vi "Drive Controller.vi"(8 "error in":errorcluster) -> ()   [LabVIEW 2018]
doc: "This VI executes continuously carrying out the current operation and responding to updates or new operation requests. It will often contain the timing or control code that is difficult to place directly in TeleOp. This VI generally opens all sensors and motors and isolates the rest of the robot code from knowing implementation details of how the operations are carried out."
uses:
  <vilib>/Rock Robotics/WPI/Framework/Completion Status.ctl
  Drive Setpoints.ctl
  Drive Operations.ctl
  <vilib>/Rock Robotics/WPI/ThirdParty/Phoenix-LabVIEW/Motor Controller/Controls/CTRE_Phoenix_MotorControl_NeutralMode.ctl
  <vilib>/Rock Robotics/WPI/ThirdParty/Phoenix-LabVIEW/Motor Controller/Controls/CTRE_Phoenix_MotorControl_ControlMode.ctl
panel:
  in  "Interactive Values":T1
  in  "Buttons":cluster{"Execute Cmd":bool, "Abort Cmd":bool}
  out "Command Timing":cluster{"Start Time (ms)":u32, "Iterations":i32}
  out "Status":T3
  out "Current\nCmd":string
  # "Tip: The graph shows the motor setpoints. It may also be helpful to observe inputs and sensor values.\nYou may also want to display tuning or debugging controls."
  # "Interactive Command: You may fill in the settings for a command\nand schedule it with the Execute button. You can observe and abort\nany command while fine tuning the code for the controller."
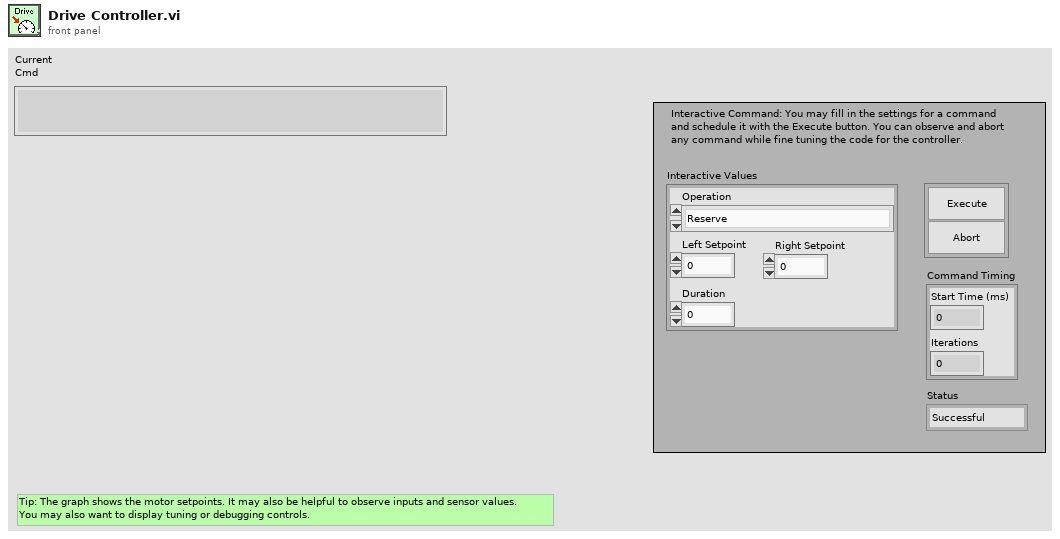
[diagram p1: front panel]
types:
  T1 = typedef "Drive Setpoints.ctl" = cluster{"Operation":T2, "Left Setpoint":dbl, "Right Setpoint":dbl, "Duration":dbl}
  T2 = typedef "Drive Operations.ctl" = enum16{"Reserve", "Read Current", "Immediate", "Drive for Time", "Drive for Distance"}
  T3 = typedef "Completion Status.ctl" = enum16{"Successful", "Aborted", "Incomplete"}
  T4 = typedef "CTRE_Phoenix_MotorControl_NeutralMode.ctl" = enum8{"EEPROMSetting", "Override to Coast", "Override to Brake"}
  T5 = enum16{"FollowerType_PercentOutput", "FollowerType_AuxOutput1"}
  T6 = typedef "WPI_MotorControlDeviceRef.ctl" = cluster{"DeviceStatus":errorcluster, "Type":T7, "PWM":cluster{"PWM Channel":T8, "DeadBand":T9}, "CAN":cluster{"Device Number":u8, "SetOutput VI Ref":variant, "GetOutput VI Ref":variant, "Enable VI Ref":variant, "Disable VI Ref":variant, "Data":variant}, "Invert":bool, "DIO PWM":cluster{"PWM \"Enable\" Channel":T8, "DIOChannel":T10, "PWM Rate":dbl}}
  T7 = typedef "WPI_MotorControlType.ctl" = enum16{"PWM", "CAN", "DIO PWM"}
  T8 = typedef "FPGA_DIOPWMChannel.ctl" = enum8{"PWM 0", "PWM 1", "PWM 2", "PWM 3", "PWM 4", "PWM 5", "PWM 6", "PWM 7", "PWM 8", "PWM 9", "PWM MXP 0", "PWM MXP 1", "PWM MXP 2", "PWM MXP 3", "PWM MXP 4", "PWM MXP 5", "PWM MXP 6", "PWM MXP 7", "PWM MXP 8", "PWM MXP 9", "Invalid"}
  T9 = typedef "WPI_PWMDeadband.ctl" = cluster{"Name":string, "maxPositivePwm":i32, "minPositivePwm":i32, "centerPwm":i32, "maxNegativePwm":i32, "minNegativePwm":i32, "angularRange":u16}
  T10 = typedef "FPGA_DIOChannel.ctl" = enum8{"DIO 0", "DIO 1", "DIO 2", "DIO 3", "DIO 4", "DIO 5", "DIO 6", "DIO 7", "DIO 8", "DIO 9", "DIO MXP 0", "DIO MXP 1", "DIO MXP 2", "DIO MXP 3", "DIO MXP 4", "DIO MXP 5", "DIO MXP 6", "DIO MXP 7", "DIO MXP 8", "DIO MXP 9", "DIO MXP 10", "DIO MXP 11", "DIO MXP 12", "DIO MXP 13", "DIO MXP 14", "DIO MXP 15", "SPI Port CS1", "SPI Port CS2", "SPI Port CS3", "SPI Port MISO", "SPI Port MOSI", "Invalid"}
  T11 = typedef "Command Status Info.ctl" = cluster{"Name":string, "Status":T3, "notifier out":T12}
  T12 = typedef "Completion Notifier.ctl" = refnum<notifier>
  T13 = cluster{"SubSystem Data":T1, cluster{"Start Time (ms)":u32, "Iterations":i32}, cluster{"Command Info":T11, "Description":string, "Default Command":T1, "queue out":refnum<queue>, "Subsystem Name":string}}
  T14 = enum16{"DemandType_Neutral", "DemandType_AuxPID", "DemandType_ArbitraryFeedForward"}
  T15 = typedef "CTRE_Phoenix_MotorControl_ControlMode.ctl" = u16
  T16 = cluster{"SubSystem Data":T1, cluster{"Start Time (ms)":u32, "Iterations":i32}, "Default Command Arguments":cluster{"Command Info":T11, "Description":string, "Default Command":T1, "queue out":refnum<queue>, "Subsystem Name":string}}
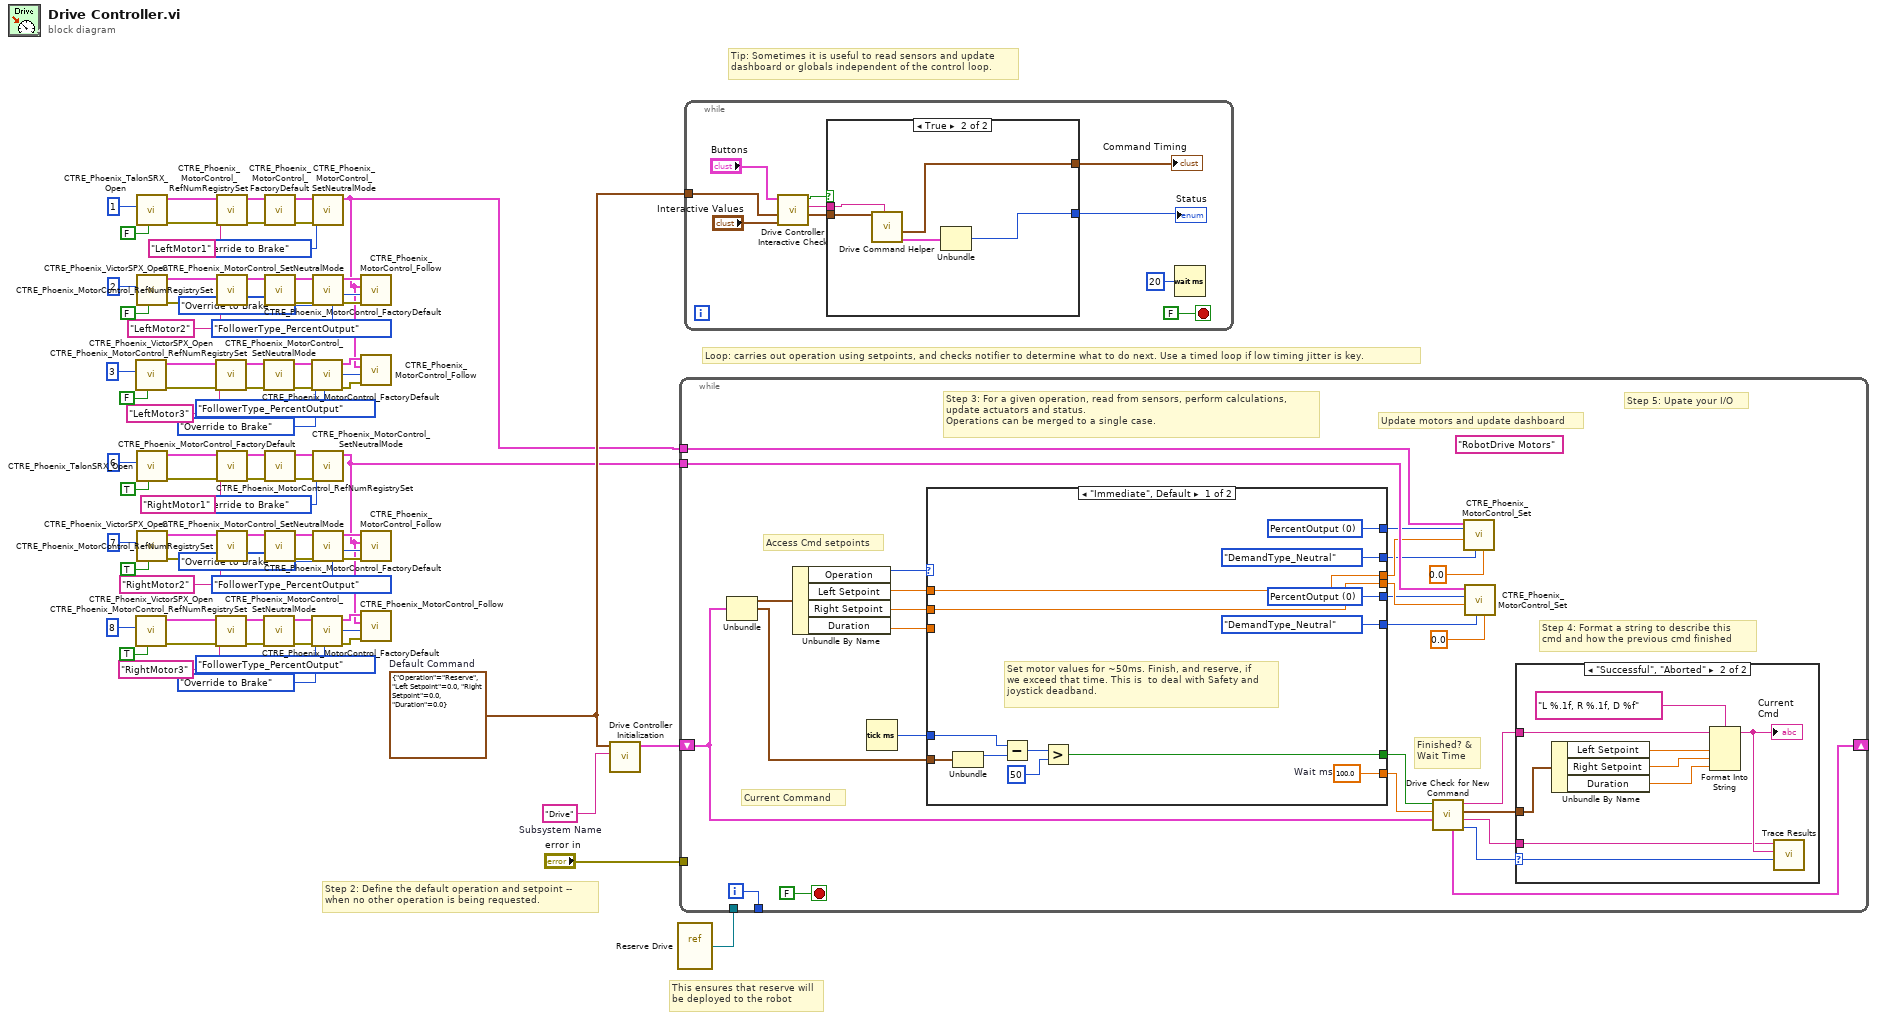
[diagram p0: block diagram]
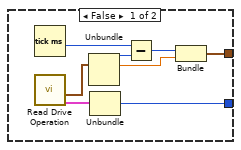
[diagram p2: hidden frame]
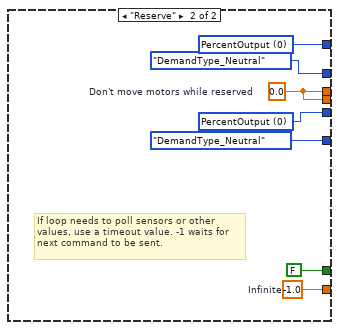
[diagram p4: hidden frame]
diagram:
  w75 = T1 {"Operation"=enum."Reserve", "Left Setpoint"=0.0, "Right Setpoint"=0.0, "Duration"=0.0}  # Default Command
  w79 = "Drive"  # Subsystem Name
  # "This ensures that reserve will\nbe deployed to the robot"
  # "Tip: Sometimes it is useful to read sensors and update\ndashboard or globals independent of the control loop."
  # "Step 2: Define the default operation and setpoint --\nwhen no other operation is being requested."
  # "Loop: carries out operation using setpoints, and checks notifier to determine what to do next. Use a timed loop if low timing jitter is key."
  n1 = call <vilib>:"CTRE_Phoenix_VictorSPX_Open.vi"("Invert"=FALSE, "Device Number"=u8 3) -> ("error out"=w48:errorcluster, "CAN Talon SRX Ref"=w49:T6)  [unwired: 8 in]
  n2 = call <vilib>:"CTRE_Phoenix_VictorSPX_Open.vi"("Invert"=TRUE, "Device Number"=u8 8) -> ("error out"=w12:errorcluster, "CAN Talon SRX Ref"=w13:T6)  [unwired: 8 in]
  n3 = call <vilib>:"CTRE_Phoenix_TalonSRX_Open.vi"("Invert"=FALSE, "Device Number"=u8 1) -> ("error out"=w68:errorcluster, "CAN Talon SRX Ref"=w74:T6)  [unwired: 8 in]
  n4 = call <vilib>:"CTRE_Phoenix_VictorSPX_Open.vi"("Invert"=FALSE, "Device Number"=u8 2) -> ("error out"=w57:errorcluster, "CAN Talon SRX Ref"=w58:T6)  [unwired: 8 in]
  n5 = call <vilib>:"CTRE_Phoenix_TalonSRX_Open.vi"("Invert"=TRUE, "Device Number"=u8 6) -> ("error out"=w32:errorcluster, "CAN Talon SRX Ref"=w38:T6)  [unwired: 8 in]
  n6 = call <vilib>:"CTRE_Phoenix_VictorSPX_Open.vi"("Invert"=TRUE, "Device Number"=u8 7) -> ("error out"=w21:errorcluster, "CAN Talon SRX Ref"=w22:T6)  [unwired: 8 in]
  n7 = call <vilib>:"CTRE_Phoenix_MotorControl_RefNumRegistrySet.vi"("error in (no error)"=w48, "refnum name"="LeftMotor3", "PhoenixMotorControlDevRef"=w49) -> ("error out"=w54:errorcluster, "PhoenixMotorControlDevRef"=w53:T6)  [unwired: 7 in]
  n8 = call <vilib>:"CTRE_Phoenix_MotorControl_RefNumRegistrySet.vi"("error in (no error)"=w12, "refnum name"="RightMotor3", "PhoenixMotorControlDevRef"=w13) -> ("error out"=w18:errorcluster, "PhoenixMotorControlDevRef"=w17:T6)  [unwired: 7 in]
  n9 = call <vilib>:"CTRE_Phoenix_MotorControl_RefNumRegistrySet.vi"("error in (no error)"=w68, "refnum name"="LeftMotor1", "PhoenixMotorControlDevRef"=w74) -> ("error out"=w70:errorcluster, "PhoenixMotorControlDevRef"=w69:T6)  [unwired: 7 in]
  n10 = call <vilib>:"CTRE_Phoenix_MotorControl_RefNumRegistrySet.vi"("error in (no error)"=w57, "refnum name"="LeftMotor2", "PhoenixMotorControlDevRef"=w58) -> ("error out"=w63:errorcluster, "PhoenixMotorControlDevRef"=w62:T6)  [unwired: 7 in]
  n11 = call <vilib>:"CTRE_Phoenix_MotorControl_RefNumRegistrySet.vi"("error in (no error)"=w32, "refnum name"="RightMotor1", "PhoenixMotorControlDevRef"=w38) -> ("error out"=w34:errorcluster, "PhoenixMotorControlDevRef"=w33:T6)  [unwired: 7 in]
  n12 = call <vilib>:"CTRE_Phoenix_MotorControl_RefNumRegistrySet.vi"("error in (no error)"=w21, "refnum name"="RightMotor2", "PhoenixMotorControlDevRef"=w22) -> ("error out"=w27:errorcluster, "PhoenixMotorControlDevRef"=w26:T6)  [unwired: 7 in]
  n13 = call <vilib>:"CTRE_Phoenix_MotorControl_FactoryDefault.vi"("error in"=w54, "PhoenixMotorControlDevRef"=w53) -> ("error out"=w52:errorcluster, "PhoenixMotorControlDevRef"=w51:T6)  [unwired: 8 in]
  n14 = call <vilib>:"CTRE_Phoenix_MotorControl_FactoryDefault.vi"("error in"=w18, "PhoenixMotorControlDevRef"=w17) -> ("error out"=w16:errorcluster, "PhoenixMotorControlDevRef"=w15:T6)  [unwired: 8 in]
  n15 = call <vilib>:"CTRE_Phoenix_MotorControl_FactoryDefault.vi"("error in"=w70, "PhoenixMotorControlDevRef"=w69) -> ("error out"=w67:errorcluster, "PhoenixMotorControlDevRef"=w66:T6)  [unwired: 8 in]
  n16 = call <vilib>:"CTRE_Phoenix_MotorControl_FactoryDefault.vi"("error in"=w63, "PhoenixMotorControlDevRef"=w62) -> ("error out"=w61:errorcluster, "PhoenixMotorControlDevRef"=w60:T6)  [unwired: 8 in]
  n17 = call <vilib>:"CTRE_Phoenix_MotorControl_FactoryDefault.vi"("error in"=w34, "PhoenixMotorControlDevRef"=w33) -> ("error out"=w31:errorcluster, "PhoenixMotorControlDevRef"=w30:T6)  [unwired: 8 in]
  n18 = call <vilib>:"CTRE_Phoenix_MotorControl_FactoryDefault.vi"("error in"=w27, "PhoenixMotorControlDevRef"=w26) -> ("error out"=w25:errorcluster, "PhoenixMotorControlDevRef"=w24:T6)  [unwired: 8 in]
  n19 = call <vilib>:"CTRE_Phoenix_MotorControl_SetNeutralMode.vi"("error in (no error)"=w52, "Motor Control Neutral Mode"=CTRE_Phoenix_MotorControl_NeutralMode."Override to Brake", "PhoenixMotorControlDevRef"=w51) -> ("error out"=w45:errorcluster, "PhoenixMotorControlDevRef"=w44:T6)  [unwired: 7 in]
  n20 = call <vilib>:"CTRE_Phoenix_MotorControl_SetNeutralMode.vi"("error in (no error)"=w16, "Motor Control Neutral Mode"=CTRE_Phoenix_MotorControl_NeutralMode."Override to Brake", "PhoenixMotorControlDevRef"=w15) -> ("error out"=w9:errorcluster, "PhoenixMotorControlDevRef"=w8:T6)  [unwired: 7 in]
  n21 = call <vilib>:"CTRE_Phoenix_MotorControl_SetNeutralMode.vi"("error in (no error)"=w67, "Motor Control Neutral Mode"=CTRE_Phoenix_MotorControl_NeutralMode."Override to Brake", "PhoenixMotorControlDevRef"=w66) -> ("PhoenixMotorControlDevRef"=w2:T6)  [unwired: 7 in, 1 out]
  n22 = call <vilib>:"CTRE_Phoenix_MotorControl_SetNeutralMode.vi"("error in (no error)"=w61, "Motor Control Neutral Mode"=CTRE_Phoenix_MotorControl_NeutralMode."Override to Brake", "PhoenixMotorControlDevRef"=w60) -> ("error out"=w47:errorcluster, "PhoenixMotorControlDevRef"=w46:T6)  [unwired: 7 in]
  n23 = call <vilib>:"CTRE_Phoenix_MotorControl_SetNeutralMode.vi"("error in (no error)"=w31, "Motor Control Neutral Mode"=CTRE_Phoenix_MotorControl_NeutralMode."Override to Brake", "PhoenixMotorControlDevRef"=w30) -> ("PhoenixMotorControlDevRef"=w1:T6)  [unwired: 7 in, 1 out]
  n24 = call <vilib>:"CTRE_Phoenix_MotorControl_SetNeutralMode.vi"("error in (no error)"=w25, "Motor Control Neutral Mode"=CTRE_Phoenix_MotorControl_NeutralMode."Override to Brake", "PhoenixMotorControlDevRef"=w24) -> ("error out"=w11:errorcluster, "PhoenixMotorControlDevRef"=w10:T6)  [unwired: 7 in]
  n25 = call <vilib>:"CTRE_Phoenix_MotorControl_Follow.vi"("error in (no error)"=w47, "FollowerType"=T5."FollowerType_PercentOutput", "Master Controller to Follow"=w2, "PhoenixMotorControlDevRef"=w46) -> ()  [unwired: 6 in, 2 out]
  n26 = call <vilib>:"CTRE_Phoenix_MotorControl_Follow.vi"("error in (no error)"=w45, "FollowerType"=T5."FollowerType_PercentOutput", "Master Controller to Follow"=w2, "PhoenixMotorControlDevRef"=w44) -> ()  [unwired: 6 in, 2 out]
  n27 = call <vilib>:"CTRE_Phoenix_MotorControl_Follow.vi"("error in (no error)"=w11, "FollowerType"=T5."FollowerType_PercentOutput", "Master Controller to Follow"=w1, "PhoenixMotorControlDevRef"=w10) -> ()  [unwired: 6 in, 2 out]
  n28 = call <vilib>:"CTRE_Phoenix_MotorControl_Follow.vi"("error in (no error)"=w9, "FollowerType"=T5."FollowerType_PercentOutput", "Master Controller to Follow"=w1, "PhoenixMotorControlDevRef"=w8) -> ()  [unwired: 6 in, 2 out]
  n29 = call "Drive Controller Initialization.vi"("Subsystem Name"=w79, "Default Command"=w75) -> ("Current Command"=w77:T13)  [unwired: 9 in]
  n30 = vi-ref "Reserve Drive.vi"() -> (w76:refnum<vi>)
  n31 = while {
    shift-right: [w97] -> _
    shift-left: w77 -> [w90]
    tunnel: [w105] -> _
    tunnel: "error in" -> [_]
    tunnel: w76 -> [_]
    tunnel: w2 -> [w89]
    tunnel: w1 -> [w88]
    i -> [w105]
    stop <- FALSE stop-if-true
    (unwired) "RobotDrive Motors" ("Name")
    # "Step 5: Upate your I/O"
    # "Step 4: Format a string to describe this\ncmd and how the previous cmd finished"
    # "Current Command"
    # "Update motors and update dashboard"
    # "Access Cmd setpoints"
    # "Finished? &\nWait Time"
    # "Step 3: For a given operation, read from sensors, perform calculations,\nupdate actuators and status.\nOperations can be merged to a single case."
    n32 = Unbundle(w90) -> ("SubSystem Data"=w104:T1, w91:cluster{"Start Time (ms)":u32, "Iterations":i32})  [unwired: 1 out]
    n33 = Unbundle By Name(w104) -> ("Operation"=w103:T2, "Left Setpoint"=w102:dbl, "Right Setpoint"=w101:dbl, "Duration"=w100:dbl)
    n34 = Tick Count (ms)() -> (millisecond timer value=w99:u32)
    n35 = case shown="\"Immediate\", Default" w103 {
      tunnel: [w128 w135] -> w96
      tunnel: [w121 FALSE ("ignore previous (F)")] -> w95
      tunnel: w91 -> [w120 _]
      tunnel: [w127 w133] -> w87
      tunnel: [w126 w133] -> w86
      tunnel: w102 -> [w127 _]
      tunnel: w101 -> [w126 _]
      tunnel: w100 -> [_ _]
      tunnel: w99 -> [w122 _]
      tunnel: [w117 w132] -> w85
      tunnel: [w119 w131] -> w84
      tunnel: [T14."DemandType_Neutral" ("DemandType") T14."DemandType_Neutral" ("DemandType")] -> w83
      tunnel: [T14."DemandType_Neutral" ("DemandType") T14."DemandType_Neutral" ("DemandType")] -> w82
      frame "Immediate", Default {
        w117 = T15 0 items=["PercentOutput"=0, "Position"=1, "Velocity"=2, "Current"=3, "Follower"=5, "MotionProfile"=6, "MotionMagic"=7, "MotionProfileArc"=10, "Disabled"=15] ("Control Mode")
        w119 = T15 0 items=["PercentOutput"=0, "Position"=1, "Velocity"=2, "Current"=3, "Follower"=5, "MotionProfile"=6, "MotionMagic"=7, "MotionProfileArc"=10, "Disabled"=15] ("Control Mode")
        w128 = 100.0  # Wait ms
        # "Set motor values for ~50ms. Finish, and reserve, if\nwe exceed that time. This is  to deal with Safety and\njoystick deadband."
        n36 = Unbundle(w120) -> ("Start Time (ms)"=w123:u32)  [unwired: 1 out]
        n37 = Subtract(x=w122, y=w123) -> (x-y=w124:u32)
        n38 = Greater?(x=w124, y=u8 50 ("Left Motor")) -> (0:w121:bool)
      }
      frame "Reserve" {
        w131 = T15 0 items=["PercentOutput"=0, "Position"=1, "Velocity"=2, "Current"=3, "Follower"=5, "MotionProfile"=6, "MotionMagic"=7, "MotionProfileArc"=10, "Disabled"=15] ("Control Mode")
        w132 = T15 0 items=["PercentOutput"=0, "Position"=1, "Velocity"=2, "Current"=3, "Follower"=5, "MotionProfile"=6, "MotionMagic"=7, "MotionProfileArc"=10, "Disabled"=15] ("Control Mode")
        w133 = 0.0  # Don't move motors while reserved
        w135 = -1.0  # Infinite
        # "If loop needs to poll sensors or other\nvalues, use a timeout value. -1 waits for\nnext command to be sent."
      }
    }
    n39 = call "Drive Check for New Command.vi"("input cluster"=w90, "Wait time (ms)"=w96, "Finished?"=w95) -> ("Completion"=w98:T3, "Subsystem Name"=w92:string, "Current Command"=w93:T1, "Initial Trace String"=w94:string, "Next Command"=w97:T16)  [unwired: 4 in]
    n40 = call <vilib>:"CTRE_Phoenix_MotorControl_Set.vi"("Demand1"=0.0, "DemandType"=w83, "Output"=w87, "Control Mode"=w84, "PhoenixMotorControlDevRef"=w89) -> ()  [unwired: 5 in, 2 out]
    n41 = call <vilib>:"CTRE_Phoenix_MotorControl_Set.vi"("Demand1"=0.0, "DemandType"=w82, "Output"=w86, "Control Mode"=w85, "PhoenixMotorControlDevRef"=w88) -> ()  [unwired: 5 in, 2 out]
    n42 = case shown="\"Successful\", \"Aborted\"" w98 {
      selector: w98 -> [_ w115]
      tunnel: w94 -> [_ w110]
      tunnel: w93 -> [_ w111]
      tunnel: w92 -> [_ w107]
      frame "Incomplete", Default {
        # "Continuing current command"
      }
      frame "Successful", "Aborted" {
        # "Report and setup for next command"
        n43 = Unbundle By Name(w111) -> ("Left Setpoint"=w113:dbl, "Right Setpoint"=w114:dbl, "Duration"=w108:dbl)
        n44 = Format Into String(format string="L %.1f, R %.1f, D %f", initial string=w110, w113, w114, w108) -> (resulting string=w109:string)  [unwired: 1 in, 1 out]
        "Current\nCmd" <- w109
        n45 = call <vilib>:"Trace Results.vi"("Status of previous command"=w115, "Description"=w109, "Subsystem"=w107) -> ()  [unwired: 9 in]
      }
    }
  }
  n46 = while {
    tunnel: w75 -> [w137]
    stop <- FALSE stop-if-true
    n47 = call "Drive Controller Interactive Check.vi"("Interactive Command In"="Interactive Values", "Default Command"=w137, "Buttons"="Buttons") -> ("Interactive Command Out"=w139:T1, "Trace String"=w140:string, "Schedule"=w141:bool)  [unwired: 6 in]
    n48 = case shown="True" w141 {
      tunnel: [w150 w158] -> w142
      tunnel: [w149 w154] -> w143
      tunnel: w140 -> [_ w156]
      tunnel: w139 -> [_ w155]
      frame False {
        n49 = Tick Count (ms)() -> (millisecond timer value=w153:u32)
        n50 = call "Read Drive Operation.vi"() -> ("Command Info"=w147:T11, "SubSystem Data"=w146:T1)  [unwired: 9 in, 1 out]
        n51 = Unbundle(w146) -> ("Operation"=w151:T2, "Left Setpoint"=w148:dbl)  [unwired: 2 out]
        n52 = Unbundle(w147) -> ("Status"=w150:T3)  [unwired: 2 out]
        n53 = Subtract(x=w153, y=w151) -> (x-y=w152:u32)
        n54 = Bundle(w152, "Left Setpoint"=w148) -> (w149:cluster{u32, "Left Setpoint":dbl})  [unwired: 1 in]
      }
      frame True {
        n55 = call "Drive Command Helper.vi"("Description"=w156, "SubSystem Data"=w155) -> ("Command Info Out"=w157:T11, "Command Timing"=w154:cluster{"Start Time (ms)":u32, "Iterations":i32})  [unwired: 7 in, 1 out]
        n56 = Unbundle(w157) -> ("Status"=w158:T3)  [unwired: 2 out]
      }
    }
    "Status" <- w142
    "Command Timing" <- w143
    n57 = Wait (ms)(milliseconds to wait=u32 20) -> ()  [unwired: 1 out]
  }
